vi "Do Request.vi"(7 "Processing In":refnum<class "Processing.lvclass">, 11 "TestQueryParamController in":refnum<class "TestQueryParamController.lvclass">) -> (0 "error out":errorcluster, 5 "Processing":refnum<class "Processing.lvclass">)   [LabVIEW 2020, in "TestQueryParamController.lvclass"]
uses:
  TestQueryParamController.lvclass
  HTTP Server/Processing/Processing.lvclass
  HTTP Server/Processing/Processing.lvclass/Processing.ctl
  Query Operation.ctl
  <vilib>/IlluminatedG/IG HTTP Utils/HTTP Utils/Request/Request.lvclass
  <vilib>/IlluminatedG/lv-stream/URI/URI.lvclass
  <vilib>/IlluminatedG/IG HTTP Utils/HTTP Utils/Response/Response.lvclass
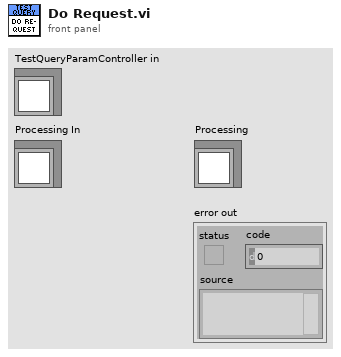
[diagram p1: front panel]
types:
  T1 = typedef "TestQueryParamController.lvclass/Query Operation.ctl" = enum16{"add", "subtract", "multiply", "divide"}
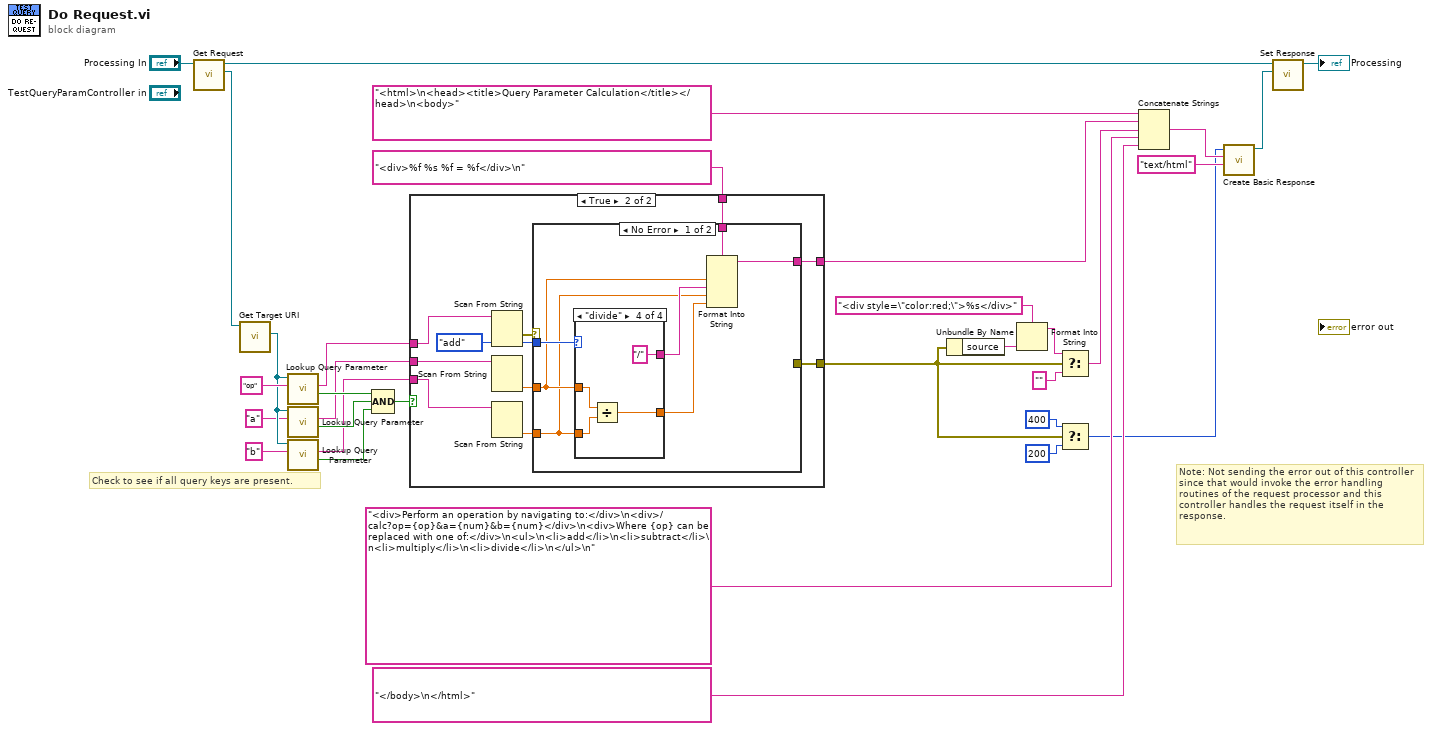
[diagram p0: block diagram]
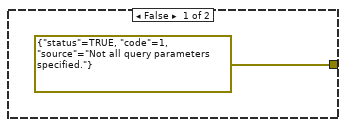
[diagram p2: hidden frame]
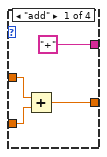
[diagram p3: hidden frame]
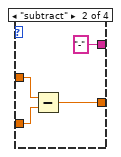
[diagram p4: hidden frame]
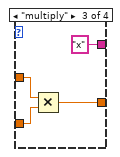
[diagram p5: hidden frame]
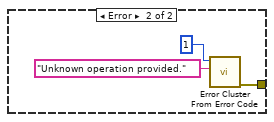
[diagram p6: hidden frame]
diagram:
  # "Note: Not sending the error out of this controller since that would invoke the error handling routines of the request processor and this controller handles the request itself in the response."
  # "Check to see if all query keys are present."
  n1 = call "Get Request.vi"("Processing in"="Processing In") -> ("Request"=w31:refnum<class "Request.lvclass">, "Processing out"=w4:refnum<class "Processing.lvclass">)  [unwired: 9 in]
  n2 = call <vilib>:"Get Target URI.vi"("Request in"=w31) -> ("Target URI"=w29:refnum<class "URI.lvclass">)  [unwired: 8 in, 2 out]
  n3 = call <vilib>:"Lookup Query Parameter.vi"("Name"="op", "URI in"=w29) -> ("Found"=w26:bool, "Value"=w20:string)  [unwired: 6 in, 2 out]
  n4 = call <vilib>:"Lookup Query Parameter.vi"("Name"="a", "URI in"=w29) -> ("Found"=w25:bool, "Value"=w21:string)  [unwired: 6 in, 2 out]
  n5 = call <vilib>:"Lookup Query Parameter.vi"("Name"="b", "URI in"=w29) -> ("Found"=w24:bool, "Value"=w22:string)  [unwired: 6 in, 2 out]
  n6 = Compound Arithmetic op=AND(w26, w25, w24) -> (w23:bool)
  n7 = case shown="True" w23 {
    tunnel: w22 -> [_ w41]
    tunnel: w21 -> [_ w42]
    tunnel: w20 -> [_ w44]
    tunnel: "<div>%f %s %f = %f</div>\n" -> [_ w36]
    tunnel: [errorcluster {"status"=TRUE, "code"=1, "source"="Not all query parameters specified."} ("error out") w35] -> w8
    tunnel: [_ w34] -> w1
    frame False {
    }
    frame True {
      n8 = Scan From String(input string=w44, default 1=Query_Operation."add" ("Query Operation")) -> (error out=w37:errorcluster, output 1=w40:T1)  [unwired: 3 in, 2 out]
      n9 = Scan From String(input string=w42) -> (output 1=w39:dbl)  [unwired: 4 in, 3 out]
      n10 = Scan From String(input string=w41) -> (output 1=w38:dbl)  [unwired: 4 in, 3 out]
      n11 = case shown="No Error" w37 {
        tunnel: w40 -> [w51 _]
        tunnel: w39 -> [w49 _]
        tunnel: w38 -> [w47 _]
        tunnel: w36 -> [w50 _]
        tunnel: [_ w68] -> w35
        tunnel: [w45 _] -> w34
        frame No Error {
          n12 = case shown="\"divide\"" w51 {
            tunnel: w47 -> [w54 w58 w62 w66]
            tunnel: w49 -> [w55 w59 w63 w67]
            tunnel: [w53 w57 w61 w65] -> w46
            tunnel: ["+" "-" "x" "/"] -> w48
            frame "add" {
              n13 = Add(x=w55, y=w54) -> (x+y=w53:dbl)
            }
            frame "subtract" {
              n14 = Subtract(x=w59, y=w58) -> (x-y=w57:dbl)
            }
            frame "multiply" {
              n15 = Multiply(x=w63, y=w62) -> (x*y=w61:dbl)
            }
            frame "divide" {
              n16 = Divide(x=w67, y=w66) -> (x/y=w65:dbl)
            }
          }
          n17 = Format Into String(format string=w50, w49, w48, w47, w46) -> (resulting string=w45:string)  [unwired: 2 in, 1 out]
        }
        frame Error {
          n18 = call <vilib>:"Error Cluster From Error Code.vi"("error message (\"\")"="Unknown operation provided." ("error message (\"\")"), "error code (0)"=1) -> ("error out"=w68:errorcluster)  [unwired: 7 in]
        }
      }
    }
  }
  n19 = Unbundle By Name(w8) -> ("source"=w17:string)
  n20 = Format Into String(format string="<div style=\"color:red;\">%s</div>", w17) -> (resulting string=w16:string)  [unwired: 2 in, 1 out]
  n21 = Select(t=w16, s=w8, f="") -> (s? t:f=w13:string)
  n22 = Select(t=u16 400 ("Status Code"), s=w8, f=u16 200 ("Status Code")) -> (s? t:f=w5:u16)
  n23 = Concatenate Strings("<html>\n<head><title>Query Parameter Calculation</title></head>\n<body>", w1, w13, "<div>Perform an operation by navigating to:</div>\n<div>/calc?op={op}&a={num}&b={num}</div>\n<div>Where {op} can be replaced with one of:</div>\n<ul>\n<li>add</li>\n<li>subtract</li>\n<li>multiply</li>\n<li>divide</li>\n</ul>\n", "</body>\n</html>") -> (w10:string)
  n24 = call <vilib>:"Create Basic Response.vi"("Content-Type (text/plain)"="text/html", "Payload"=w10, "Status Code"=w5) -> ("Response out"=w2:refnum<class "Response.lvclass">)  [unwired: 7 in, 1 out]
  n25 = call "Set Response.vi"("Response"=w2, "Processing in"=w4) -> ("Processing out"=→"Processing":refnum<class "Processing.lvclass">)  [unwired: 9 in]
